vi "Flatten UIP Value.vi"(11 "Visible UIP In":refnum<class "VisibleUIP.lvclass">) -> (0 "Error Out":errorcluster, 2 "String Value":string, 3 "Visible UIP Out":refnum<class "VisibleUIP.lvclass">)   [LabVIEW 2015, in "VisibleUIP.lvclass"]
uses:
  VisibleUIP.lvclass
  VisibleUIP.lvclass/VisibleUIP.ctl
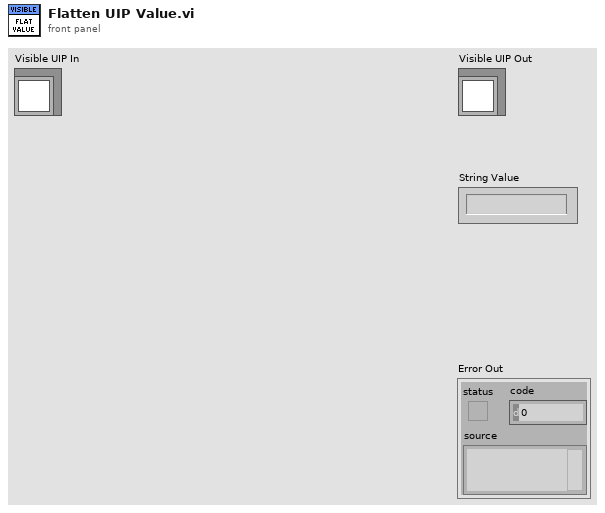
[diagram p1: front panel]
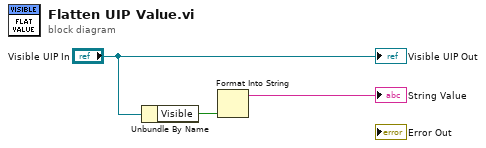
[diagram p0: block diagram]
diagram:
  n1 = Unbundle By Name("Visible UIP In") -> ("Visible"=w2:bool)
  n2 = Format Into String(w2) -> (resulting string=→"String Value":string)  [unwired: 3 in, 1 out]
  "Visible UIP Out" <- "Visible UIP In"
